vi "FakeCameraAndMotors.vi"() -> ()   [LabVIEW 2011]
uses:
  <vilib>/vision/Image Controls.llb/IMAQ Image.ctl
  BeadTracker2.llb/CmdEnum_CameraIn.ctl
  BeadTracker2.llb/CmdData_SetMotorPos.ctl
  BeadTracker2.llb/MotorPosType.ctl
  BeadTracker2.llb/XYf.ctl
  BeadTracker2.llb/MotorPosFlagsType.ctl
  BeadTracker2.llb/CmdData_GrabParams.ctl
  qtrk/QTrk.llb/QTrkInstance.ctl
  BeadTracker2.llb/CmdData_NewFrame.ctl
  BeadTracker2.llb/CmdEnum_CameraFrameType.ctl
  qtrk/QTrk.llb/QTrkZCommandType.ctl
  BeadTracker2.llb/GlobalVariables.vi
  qtrk/QTrk.llb/QTrkDLL.vi
panel:
  out "max value":sgl
  out "Image View":T1(plugin-control)
  in  "Image":T1
  in  "Image parameters":T2={"Width"=80, "Height"=80, "position"={"x"=40.0, "y"=40.0}, "magnification"=1.0, "LUT radii"={"min"=0.0, "max"=40.0}}
  in  "LUT (in)":dbl[][](graph)=array200x64[12800 elements]
  in  "Update image?":bool
  in  "Position.Piezo Z":dbl(slide) scale=0.0..100.0
  in  "FPS":u32=100
  in  "Camera Init":bool
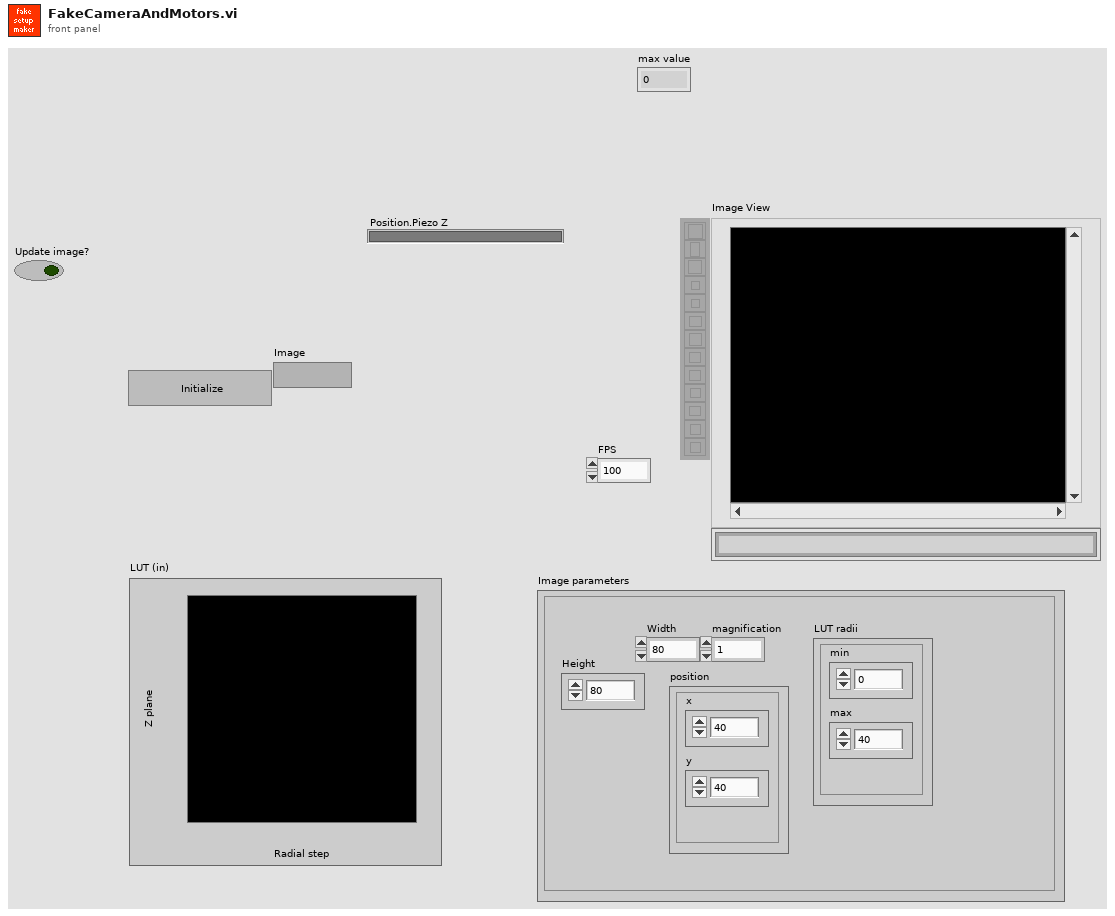
[diagram p1: front panel]
types:
  T1 = typedef "IMAQ Image.ctl" = refnum<image>
  T2 = cluster{"Width":i32, "Height":i32, "position":cluster{"x":sgl, "y":sgl}, "magnification":sgl, "LUT radii":cluster{"min":sgl, "max":sgl}}
  T3 = typedef "QueueListType.ctl" = cluster{"Motor In":refnum<queue>, "User Interface Image View":refnum<queue>, "Camera In":refnum<queue>, "User Interface Event Notifier":refnum<notifier>, "Initialized?":bool}
  T4 = typedef "CmdData_SetMotorPos.ctl" = cluster{"Position":T5, "Move flags":T7, "Speed":T5, "Instant?":bool}
  T5 = typedef "MotorPosType.ctl" = cluster{"Magnet Z":dbl, "Magnet rotation":dbl, "Camera":T6, "Piezo XY":T6, "Piezo Z":dbl}
  T6 = typedef "XYf.ctl" = cluster{"X":sgl, "Y":sgl}
  T7 = typedef "MotorPosFlagsType.ctl" = cluster{"Magnet Z":bool, "Magnet rotation":bool, "Camera":cluster{"X":bool, "Y":bool}, "Piezo XY":cluster{"X":bool, "Y":bool}, "Piezo Z":bool}
  T8 = typedef "Cmd_MotorIn.ctl" = cluster{"Command Type":T9, "Msg Data":variant}
  T9 = typedef "CmdEnum_MotorIn.ctl" = enum32{"Init", "Close", "SetPosition", "UpdatePositions"}
  T10 = typedef "MotorStateType.ctl" = cluster{"Enabled?":bool, "Current Position":T5, "Update counter":i32}
  T11 = typedef "CmdEnum_CameraIn.ctl" = enum32{"Init", "Close", "ShowSettingsDialog", "EndGrab", "GrabZLUT", "GrabToTracker", "GrabToQueue", "AdjustROIs"}
  T12 = typedef "CmdData_GrabParams.ctl" = cluster{"QTrk Instance":T13, "Output Queue":refnum<queue>}
  T13 = typedef "QTrkInstance.ctl" = cluster{"QTrk Pointer":u64}
  T14 = typedef "CmdData_NewFrame.ctl" = cluster{"Buffer Image":T1, "Frame #":i32, "Hardware ROI Index":i32, "Timestamp":dbl, "Type":T15}
  T15 = typedef "CmdEnum_CameraFrameType.ctl" = enum16{"Full", "HardwareROI", "EndGrabMarker"}
  T16 = typedef "QTrkZCommandType.ctl" = enum16{"Nothing", "ComputeZ", "BuildZLUT"}
  T17 = typedef "Cmd_CameraIn.ctl" = cluster{"ID":T11, "Msg Data":variant}
  T18 = typedef "MeasureConfigType.ctl" = cluster{"Bead locations":cluster{"X":i32, "Y":i32}[], "ROI":i32, "Experiment base path":path, "Image output subdir":string, "Output mode":T19, "Traces output subdir":string, "QTrk Settings":T20, "Tracking Config":cluster{"Number of steps":i32, "ZLUT stepsize (um)":sgl, "Z correction factor":sgl, "Start piezo Z (um)":sgl, "Pixel size (nm)":sgl}, "Experiment Name":string, "Program":T21, "ZLUT":sgl[][][], "Camera settings":variant, "Experiment Script":string, "2D Localization Type":T25, "Max frames in memory":i32, "Save traces as binary":bool, "Pixel Calibration Gain Image":string, "Pixel Calibration Offset Image":string, "Use pixel calibration images":bool}
  T19 = typedef "MeasureConfigOutputMode.ctl" = enum16{"None", "Track", "SaveImages"}
  T20 = typedef "QTrkSettings.ctl" = cluster{"Image width":i32, "Image height":i32, "Number of threads (CPU based)":i32, "CUDA Device":i32, "COM Background correction factor":sgl, "Gaussian 2D Fit Iterations":i32, "ZLUT MinRadius":sgl, "ZLUT Radial Coverage":sgl, "ZLUT Angular Coverage":sgl, "ZLUT ROI Coverage":sgl, "QI Iterations":i32, "QI MinRadius":sgl, "QI Radial Coverage":sgl, "QI Angular Coverage":sgl, "QI ROI Coverage":sgl, "QI Angular Step \nIteration Factor":sgl, "XCOR Profile Length":i32, "XCOR Profile Width":i32, "XCOR Iterations":i32}
  T21 = typedef "ExperimentProgramType.ctl" = cluster{"Commands":T22[], "Motor Axis accuracy conditions":T5, "Axis flags":T7}
  T22 = typedef "ExProgCommandType.ctl" = cluster{"cmd":T23, "axis":T24, "value/pos":dbl, "speed":dbl, "name":string}
  T23 = typedef "ExProgCommandEnumType.ctl" = enum16{"wait", "move", "acquire", "idle", "rmove", "when", "section", "stop"}
  T24 = typedef "MotorAxisEnum.ctl" = enum16{"no axis", "magrot", "magpos", "px", "py", "pz", "camx", "camy"}
  T25 = typedef "QTrkLocalizationType.ctl" = enum16{"Center-of-Mass", "1D Cross-Correlation", "Quadrant Interpolation"}
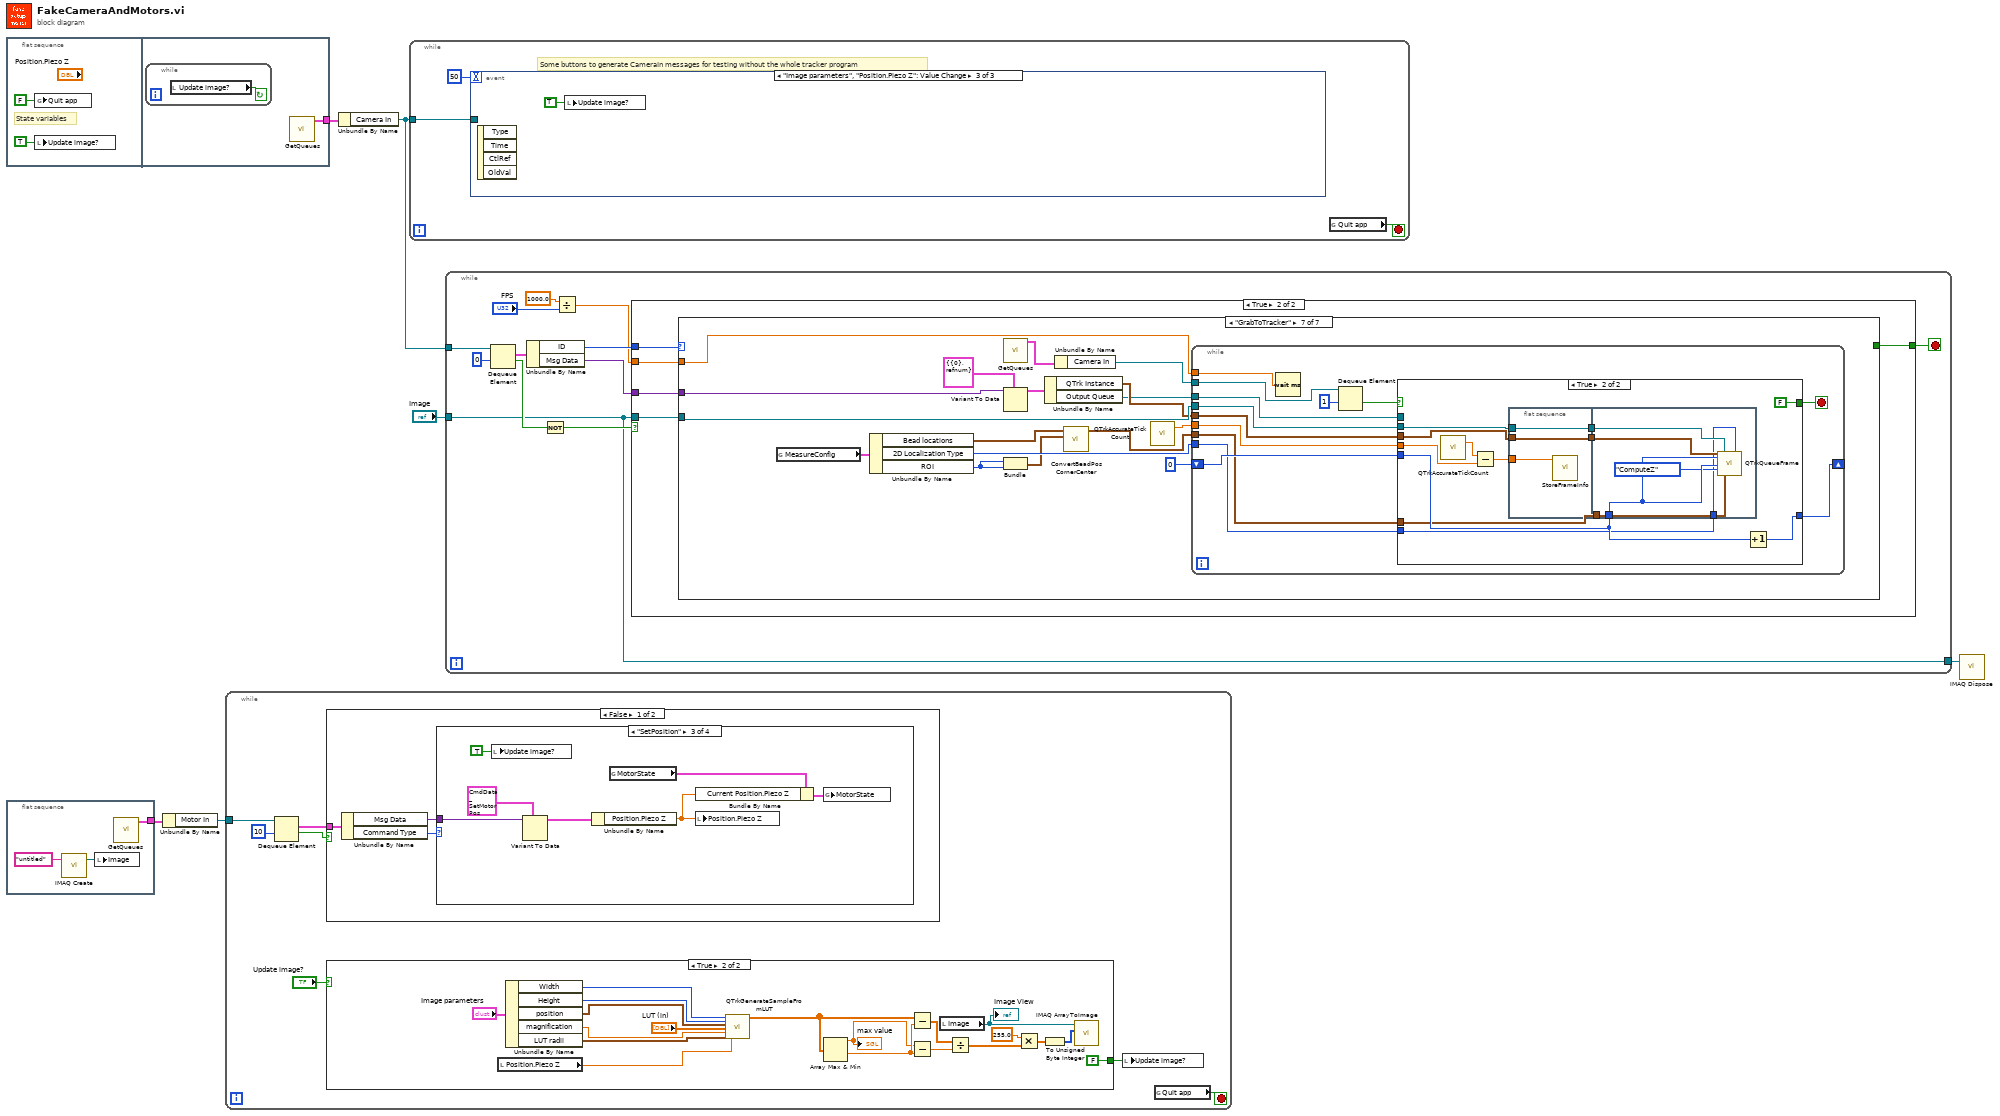
[diagram p0: block diagram]
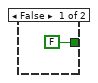
[diagram p2: hidden frame]
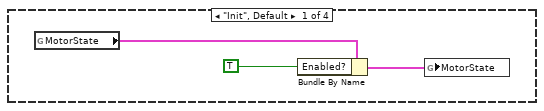
[diagram p3: hidden frame]
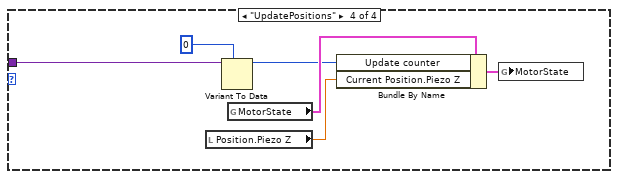
[diagram p5: hidden frame]
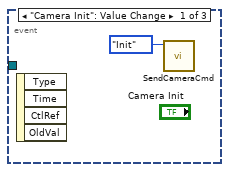
[diagram p7: hidden frame]
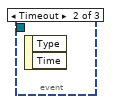
[diagram p8: hidden frame]
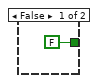
[diagram p9: hidden frame]
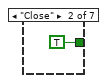
[diagram p11: hidden frame]
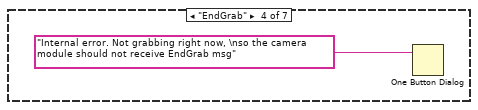
[diagram p13: hidden frame]
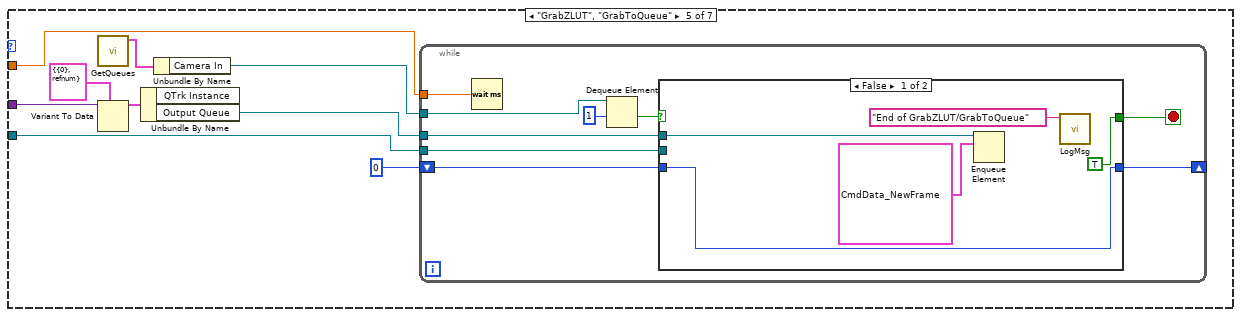
[diagram p14: hidden frame]
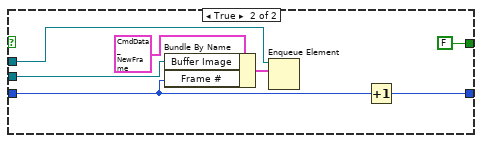
[diagram p15: hidden frame]
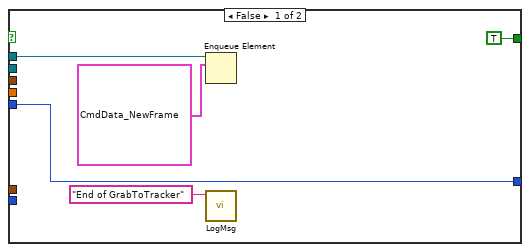
[diagram p17: hidden frame]
diagram:
  n1 = flat-sequence {
    tunnel: [w9] -> w5
    frame #0 {
      # "State variables"
      n2 = global write "GlobalVariables.vi" "Quit app"(FALSE ("Quit app")) -> ()
      n3 = local write "Update image?"(TRUE ("Update image?")) -> ()
    }
    frame #1 {
      n4 = while {
        stop <- w10 continue-if-true
        n5 = local read "Update image?"() -> (w10:bool)
      }
      n6 = call "GetQueues.vi"() -> ("Queue List"=w9:T3)  [unwired: 10 in, 1 out]
    }
  }
  n7 = flat-sequence {
    tunnel: [w11] -> w1
    frame #0 {
      n8 = call "IMAQ Create"("Image Name"="untitled") -> ("New Image"=w13:T1)  [unwired: 4 in, 1 out]
      n9 = local write "Image"(w13) -> ()
      n10 = call "GetQueues.vi"() -> ("Queue List"=w11:T3)  [unwired: 10 in, 1 out]
    }
  }
  n11 = Unbundle By Name(w1) -> ("Motor In"=w3:refnum<queue>)
  n12 = while {
    tunnel: w3 -> [w19]
    stop <- w20 stop-if-true
    n13 = Dequeue Element(queue=w19, timeout in ms (-1)=10) -> (element=w16:T8, timed out?=w17:bool)  [unwired: 1 in, 2 out]
    n14 = case shown="False" w17 {
      tunnel: w16 -> [w43 _]
      frame False {
        n15 = Unbundle By Name(w43) -> ("Msg Data"=w41:variant, "Command Type"=w42:T9)
        n16 = case shown="\"SetPosition\"" w42 {
          tunnel: w41 -> [_ _ w53 w58]
          frame "Init", Default {
            n17 = global read "GlobalVariables.vi" "MotorState"() -> (w46:T10)
            n18 = Bundle By Name(cluster=w46, "Enabled?"=TRUE) -> (w45:T10)
            n19 = global write "GlobalVariables.vi" "MotorState"(w45) -> ()
          }
          frame "Close" {
          }
          frame "SetPosition" {
            n20 = local write "Update image?"(TRUE ("Update image?")) -> ()
            n21 = Variant To Data(type=T4 {"Position"={"Magnet Z"=0.0, "Magnet rotation"=0.0, "Camera"={"X"=0.0, "Y"=0.0}, "Piezo XY"={"X"=0.0, "Y"=0.0}, "Piezo Z"=0.0}, "Move flags"={"Magnet Z"=FALSE, "Magnet rotation"=FALSE, "Camera"={"X"=FALSE, "Y"=FALSE}, "Piezo XY"={"X"=FALSE, "Y"=FALSE}, "Piezo Z"=FALSE}, "Speed"={"Magnet Z"=0.0, "Magnet rotation"=0.0, "Camera"={"X"=0.0, "Y"=0.0}, "Piezo XY"={"X"=0.0, "Y"=0.0}, "Piezo Z"=0.0}, "Instant?"=FALSE} ("SetMotorPosCmdData"), Variant=w53) -> (data=w51:T4)  [unwired: 1 in, 1 out]
            n22 = Unbundle By Name(w51) -> ("Position.Piezo Z"=w48:dbl)
            n23 = global read "GlobalVariables.vi" "MotorState"() -> (w50:T10)
            n24 = Bundle By Name(cluster=w50, "Current Position.Piezo Z"=w48) -> (w49:T10)
            n25 = local write "Position.Piezo Z"(w48) -> ()
            n26 = global write "GlobalVariables.vi" "MotorState"(w49) -> ()
          }
          frame "UpdatePositions" {
            n27 = local read "Position.Piezo Z"() -> (w55:dbl)
            n28 = Variant To Data(type=0 ("timeout in ms (-1)"), Variant=w58) -> (data=w56:i32)  [unwired: 1 in, 1 out]
            n29 = global read "GlobalVariables.vi" "MotorState"() -> (w59:T10)
            n30 = Bundle By Name(cluster=w59, "Update counter"=w56, "Current Position.Piezo Z"=w55) -> (w54:T10)
            n31 = global write "GlobalVariables.vi" "MotorState"(w54) -> ()
          }
        }
      }
      frame True {
      }
    }
    n32 = case shown="True" "Update image?" {
      tunnel: [FALSE ("Update image?") FALSE ("Update image?")] -> w14
      frame False {
      }
      frame True {
        n33 = local read "Position.Piezo Z"() -> (w39:dbl)
        n34 = Unbundle By Name("Image parameters") -> ("Width"=w37:i32, "Height"=w36:i32, "position"=w35:cluster{"x":sgl, "y":sgl}, "magnification"=w34:sgl, "LUT radii"=w33:cluster{"min":sgl, "max":sgl})
        n35 = call "QTrkGenerateSampleFromLUT.vi"("Width"=w37, "Height"=w36, "position"=w35, "LUT"="LUT (in)", "magnification"=w34, "LUT radii"=w33, "z"=w39) -> ("image"=w22:sgl[][])  [unwired: 12 in]
        n36 = Array Max & Min(array=w22) -> (max value=w31:sgl, min value=w32:sgl)  [unwired: 2 out]
        "max value" <- w31
        n37 = Subtract(x=w22, y=w32) -> (x-y=w30:sgl[][])
        n38 = Subtract(x=w31, y=w32) -> (x-y=w29:sgl)
        n39 = local read "Image"() -> (w23:T1)
        "Image View" <- w23
        n40 = Divide(x=w30, y=w29) -> (x/y=w28:sgl[][])
        n41 = Multiply(x=sgl 255.0, y=w28) -> (x*y=w26:sgl[][])
        n42 = To Unsigned Byte Integer(number=w26) -> (unsigned 8bit integer=w25:u8[][])
        n43 = call "IMAQ ArrayToImage"("Image Pixels (U8)"=w25, "Image"=w23) -> ()  [unwired: 8 in, 2 out]
      }
    }
    n44 = local write "Update image?"(w14) -> ()
    n45 = global read "GlobalVariables.vi" "Quit app"() -> (w20:bool)
  }
  n46 = Unbundle By Name(w5) -> ("Camera In"=w6:refnum<queue>)
  n47 = while {
    tunnel: w6 -> [w60]
    stop <- w61 stop-if-true
    # "Some buttons to generate CameraIn messages for testing without the whole tracker program"
    n48 = event shown="[2] \"Image parameters\", \"Position.Piezo Z\": Value Change" {
      selector: _ -> [_ _ _]
      dyn-events: _ -> [_ _ _]
      timeout: 50 -> [_ _ _]
      tunnel: w60 -> [_ _ _]
      event "Camera Init": Value Change {
        n49 = event-data() -> ()  [unwired: 1 in, 4 out]
        n50 = call "SendCameraCmd.vi"("Camera cmd (SettingsDlg)"=CmdEnum_CameraIn."Init" ("Command Type")) -> ()  [unwired: 11 in]
      }
      event Timeout {
        n51 = event-data() -> ()  [unwired: 1 in, 2 out]
      }
      event "Image parameters", "Position.Piezo Z": Value Change {
        n52 = event-data() -> ()  [unwired: 1 in, 4 out]
        n53 = local write "Update image?"(TRUE ("Update image?")) -> ()
      }
    }
    n54 = global read "GlobalVariables.vi" "Quit app"() -> (w61:bool)
  }
  n55 = while {
    tunnel: w6 -> [w76]
    tunnel: "Image" -> [w65]
    tunnel: [w65] -> w4
    stop <- w70 stop-if-true
    n56 = Dequeue Element(queue=w76, timeout in ms (-1)=0) -> (element=w72:T17, timed out?=w75:bool)  [unwired: 1 in, 2 out]
    n57 = Unbundle By Name(w72) -> ("ID"=w71:T11, "Msg Data"=w69:variant)
    n58 = Not(x=w75) -> (.not. x?=w74:bool)
    n59 = Divide(x=1000.0, y="FPS") -> (x/y=w66:dbl)
    n60 = case shown="True" w74 {
      tunnel: w71 -> [_ w82]
      tunnel: [FALSE w81] -> w70
      tunnel: w69 -> [_ w80]
      tunnel: w65 -> [_ w79]
      tunnel: w66 -> [_ w78]
      frame False {
      }
      frame True {
        n61 = case shown="\"GrabToTracker\"" w82 {
          tunnel: [_ TRUE _ _ _ _ _] -> w81
          tunnel: w80 -> [_ _ _ _ w86 _ w125]
          tunnel: w79 -> [_ _ _ _ w87 _ w126]
          tunnel: w78 -> [_ _ _ _ w85 _ w121]
          frame "Init", Default {
          }
          frame "Close" {
          }
          frame "ShowSettingsDialog" {
          }
          frame "EndGrab" {
            n62 = One Button Dialog(message="Internal error. Not grabbing right now, \nso the camera module should not receive EndGrab msg") -> ()  [unwired: 1 in, 1 out]
          }
          frame "GrabZLUT", "GrabToQueue" {
            n63 = call "GetQueues.vi"() -> ("Queue List"=w91:T3)  [unwired: 10 in, 1 out]
            n64 = Variant To Data(type=T12 {"QTrk Instance"={"QTrk Pointer"=0}, "Output Queue"=refnum} ("GrabSessionParameters"), Variant=w86) -> (data=w92:T12)  [unwired: 1 in, 1 out]
            n65 = Unbundle By Name(w92) -> ("Output Queue"=w89:refnum<queue>)  [unwired: 1 out]
            n66 = Unbundle By Name(w91) -> ("Camera In"=w90:refnum<queue>)
            n67 = while {
              tunnel: w90 -> [w102]
              tunnel: w87 -> [w98]
              tunnel: w89 -> [w97]
              shift-right: [w95] -> _
              shift-left: 0 ("Frame #") -> [w96]
              tunnel: w85 -> [w94]
              stop <- w99 stop-if-true
              n68 = Wait (ms)(milliseconds to wait=w94) -> ()  [unwired: 1 out]
              n69 = Dequeue Element(queue=w102, timeout in ms (-1)=1) -> (timed out?=w100:bool)  [unwired: 1 in, 3 out]
              n70 = case shown="False" w100 {
                tunnel: [TRUE FALSE] -> w99
                tunnel: w98 -> [_ w110]
                tunnel: w97 -> [w103 w113]
                tunnel: w96 -> [w106 w109]
                tunnel: [w106 w108] -> w95
                frame False {
                  n71 = Enqueue Element(queue=w103, element=T14 {"Buffer Image"=refnum, "Frame #"=0, "Hardware ROI Index"=0, "Timestamp"=0.0, "Type"=enum."EndGrabMarker"}) -> ()  [unwired: 2 in, 3 out]
                  n72 = call "LogMsg.vi"("msg"="End of GrabZLUT/GrabToQueue") -> ()  [unwired: 11 in]
                }
                frame True {
                  n73 = Bundle By Name(cluster=T14 {"Buffer Image"=refnum, "Frame #"=0, "Hardware ROI Index"=0, "Timestamp"=0.0, "Type"=enum."Full"} ("element"), "Buffer Image"=w110, "Frame #"=w109) -> (w111:T14)
                  n74 = Enqueue Element(queue=w113, element=w111) -> ()  [unwired: 2 in, 3 out]
                  n75 = Increment(x=w109) -> (x+1=w108:i32)
                }
              }
            }
          }
          frame "AdjustROIs" {
          }
          frame "GrabToTracker" {
            n76 = global read "GlobalVariables.vi" "MeasureConfig"() -> (w123:T18)
            n77 = Unbundle By Name(w123) -> ("Bead locations"=w119:cluster{"X":i32, "Y":i32}[], "2D Localization Type"=w122:T25, "ROI"=w117:i32)
            n78 = call "GetQueues.vi"() -> ("Queue List"=w129:T3)  [unwired: 10 in, 1 out]
            n79 = Variant To Data(type=T12 {"QTrk Instance"={"QTrk Pointer"=0}, "Output Queue"=refnum} ("GrabSessionParameters"), Variant=w125) -> (data=w130:T12)  [unwired: 1 in, 1 out]
            n80 = Bundle("ROI"=w117, "ROI"=w117) -> (w118:cluster{"ROI":i32, "ROI":i32})  [unwired: 1 in]
            n81 = Unbundle By Name(w130) -> ("QTrk Instance"=w124:T13, "Output Queue"=w120:refnum<queue>)
            n82 = Unbundle By Name(w129) -> ("Camera In"=w128:refnum<queue>)
            n83 = call "ConvertBeadPosCornerCenter.vi"("ROI Size"=w118, "Center-based bead locations"=w119) -> ("Corner-based bead pos (out)"=w116:cluster{"X":i32, "Y":i32}[])  [unwired: 8 in, 1 out]
            n84 = call "QTrkAccurateTickCount.vi"() -> ("tick count (ms)"=w115:dbl)  [unwired: 2 in, 1 out]
            n85 = while {
              tunnel: w128 -> [w144]
              tunnel: w126 -> [w140]
              shift-right: [w138] -> _
              shift-left: 0 ("Frame #") -> [w139]
              tunnel: w124 -> [w137]
              tunnel: w122 -> [w136]
              tunnel: w121 -> [w135]
              tunnel: w120 -> [w134]
              tunnel: w116 -> [w133]
              tunnel: w115 -> [w132]
              stop <- w141 stop-if-true
              n86 = Wait (ms)(milliseconds to wait=w135) -> ()  [unwired: 1 out]
              n87 = Dequeue Element(queue=w144, timeout in ms (-1)=1) -> (timed out?=w142:bool)  [unwired: 1 in, 3 out]
              n88 = case shown="True" w142 {
                tunnel: [TRUE FALSE] -> w141
                tunnel: w140 -> [_ w157]
                tunnel: w139 -> [w148 w158]
                tunnel: [w148 w160] -> w138
                tunnel: w137 -> [_ w159]
                tunnel: w136 -> [_ w156]
                tunnel: w134 -> [w145 _]
                tunnel: w133 -> [_ w155]
                tunnel: w132 -> [_ w153]
                frame False {
                  n89 = Enqueue Element(queue=w145, element=T14 {"Buffer Image"=refnum, "Frame #"=0, "Hardware ROI Index"=0, "Timestamp"=0.0, "Type"=enum."EndGrabMarker"}) -> ()  [unwired: 2 in, 3 out]
                  n90 = call "LogMsg.vi"("msg"="End of GrabToTracker") -> ()  [unwired: 11 in]
                }
                frame True {
                  n91 = call "QTrkAccurateTickCount.vi"() -> ("tick count (ms)"=w154:dbl)  [unwired: 2 in, 1 out]
                  n92 = Subtract(x=w154, y=w153) -> (x-y=w150:dbl)
                  n93 = flat-sequence {
                    tunnel: w157 -> [w163]
                    tunnel: w159 -> [w164]
                    tunnel: [w164] -> w152
                    tunnel: [w163] -> w151
                    tunnel: w150 -> [w162]
                    tunnel: w158 -> [w169]
                    tunnel: w156 -> [w166]
                    tunnel: w155 -> [w165]
                    tunnel: w152 -> [w170]
                    tunnel: w151 -> [w167]
                    frame #0 {
                      n94 = call "StoreFrameInfo.vi"("Timestamp"=w162) -> ()  [unwired: 11 in]
                    }
                    frame #1 {
                      n95 = call "QTrkQueueFrame.vi"("QTrk Instance"=w170, "frame#"=w169, "timestamp"=w169, "Z Command (None)"=QTrkZCommandType."ComputeZ", "Image"=w167, "ROI Positions (corner-based)"=w165, "2D Localization Type (COM)"=w166) -> ()  [unwired: 10 in, 3 out]
                    }
                  }
                  n96 = Increment(x=w158) -> (x+1=w160:i32)
                }
              }
            }
          }
        }
      }
    }
  }
  n97 = call "IMAQ Dispose"("Image"=w4) -> ()  [unwired: 5 in, 1 out]
